vi "xPack (SubVI).vi"(9 "ValueArray":i32[](array[numeric]), 10 "AddrArray":i32[](array[numeric]), 11 "cmd":string) -> (2 "String":string, 3 "size(s)":i32)   [LabVIEW 2018]
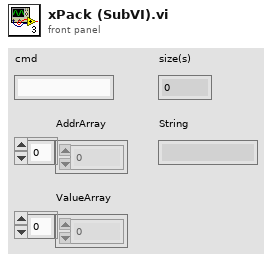
[diagram p1: front panel]
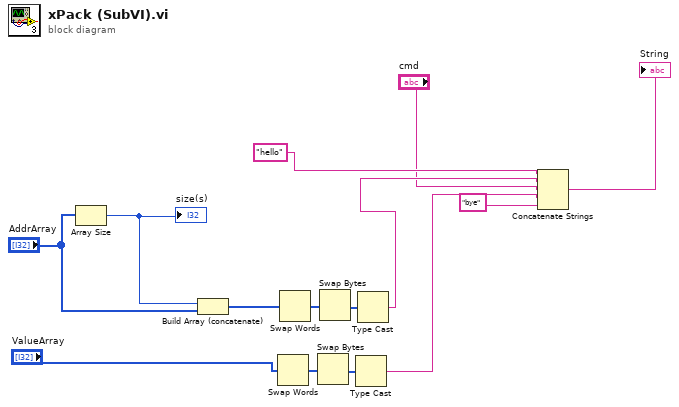
[diagram p0: block diagram]
diagram:
  n1 = Array Size(array="AddrArray") -> (size(s)=w8:i32)
  "size(s)" <- w8
  n2 = Build Array (concatenate)(w8, "AddrArray") -> (w11:i32[])
  n3 = Swap Words(1:"ValueArray") -> (0:w7:i32[])
  n4 = Swap Words(1:w11) -> (0:w9:i32[])
  n5 = Swap Bytes(anything=w7) -> (byte swapped=w6:i32[])
  n6 = Swap Bytes(anything=w9) -> (byte swapped=w10:i32[])
  n7 = Type Cast(x=w6) -> (*(type *) &x=w2:string)  [unwired: 1 in]
  n8 = Type Cast(x=w10) -> (*(type *) &x=w4:string)  [unwired: 1 in]
  n9 = Concatenate Strings("hello", w4, "cmd", w2, "bye" ("element")) -> (→"String":string)
